vi "Parse Numbers.vi"(11 "Card":string) -> (2 "set":set{string}(c389), 3 "string array":string[](array[string]))   [LabVIEW 2020, in "Card.lvclass"]
uses:
  Card.lvclass
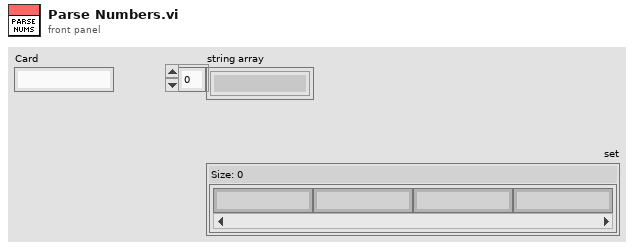
[diagram p1: front panel]
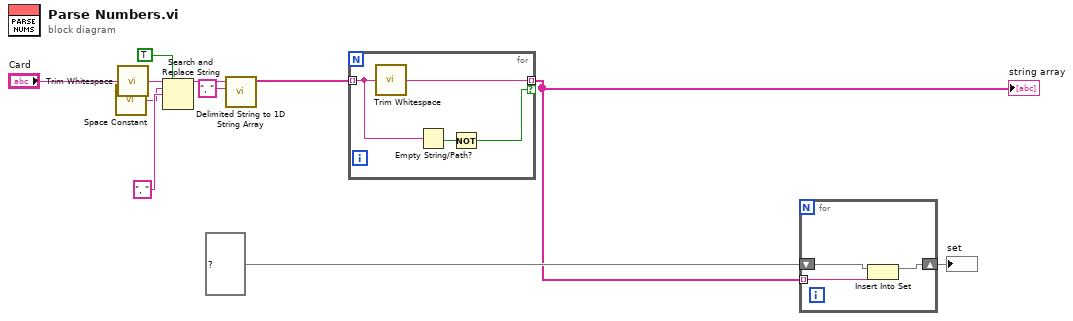
[diagram p0: block diagram]
diagram:
  n1 = call <vilib>:"Space Constant.vi"() -> ("String"=w8:string)
  n2 = call <vilib>:"Trim Whitespace.vi"("string"="Card") -> ("trimmed string"=w6:string)  [unwired: 1 in]
  n3 = Search and Replace String(replace all?=TRUE ("replace all? (F)"), input string=w6, search string=w8, replace string=", " ("replace string (\"\")")) -> (result string=w10:string)  [unwired: 4 in, 3 out]
  n4 = call <vilib>:"Delimited String to 1D String Array.vi"("delimiter"=", ", "delimited string"=w10) -> ("string array"=w3:string[])  [unwired: 9 in]
  n5 = for {
    tunnel: w3 -> [w14] mode=indexing
    tunnel: [w15] -> w1 mode=indexing if=w12
    n6 = call <vilib>:"Trim Whitespace.vi"("string"=w14) -> ("trimmed string"=w15:string)  [unwired: 1 in]
    n7 = Empty String/Path?(string/path=w14) -> (empty?=w13:bool)
    n8 = Not(x=w13) -> (.not. x?=w12:bool)
  }
  "string array" <- w1
  n9 = for {
    shift-right: [w17] -> w2
    shift-left: set{string} {} ("set") -> [w18]
    tunnel: w1 -> [w16] mode=indexing
    n10 = Insert Into Set(10:w16, 11:w18) -> (3:w17:set{string})  [unwired: 1 out]
  }
  "set" <- w2
